vi "test Loopback MC.vi"(8 "error in":errorcluster, 11 "TestCase in":refnum<class "Loopback.lvclass">) -> (0 "error out":errorcluster, 3 "TestCase out":refnum<class "Loopback.lvclass">)   [LabVIEW 2020, in "Loopback.lvclass"]
uses:
  Loopback.lvclass
  C:/dev/niveristand-custom-device-testing-tools/VeriStandTestCase/VeriStandTestCase.lvclass
  <vilib>/numeric/Random Number (Range) U64.vi
  485b7c2b-8320-4722-9ec7-d01f27c65546.vi
  0f9dda61-2c21-4955-8588-a8fc95227647.vi
  <vilib>/numeric/sub_Random U32.vi
  <vilib>/NI VeriStand/Execution/Workspace/NI VeriStand - Set Single Channel Value.vi
  <vilib>/NI VeriStand/Execution/Workspace/NI VeriStand - Get Single Channel Value.vi
  <vilib>/addons/_JKI Toolkits/VI Tester/TestCase.llb/TestCase.lvclass
  <vilib>/NI VeriStand/Execution/Workspace/NI_VS Workspace ExecutionAPI.lvlib
  C:/Program Files (x86)/National Instruments/LabVIEW 2020/vi.lib/addons/_JKI Toolkits/VI Tester/TestCase.llb/TestCase.lvclass
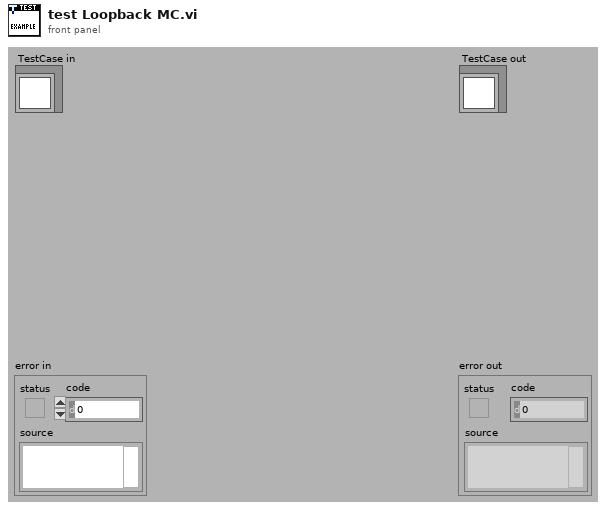
[diagram p1: front panel]
types:
  T1 = typedef "NI_VS Workspace ExecutionAPI.lvlib/WorkspaceAPI.ctl" = refnum<k24>
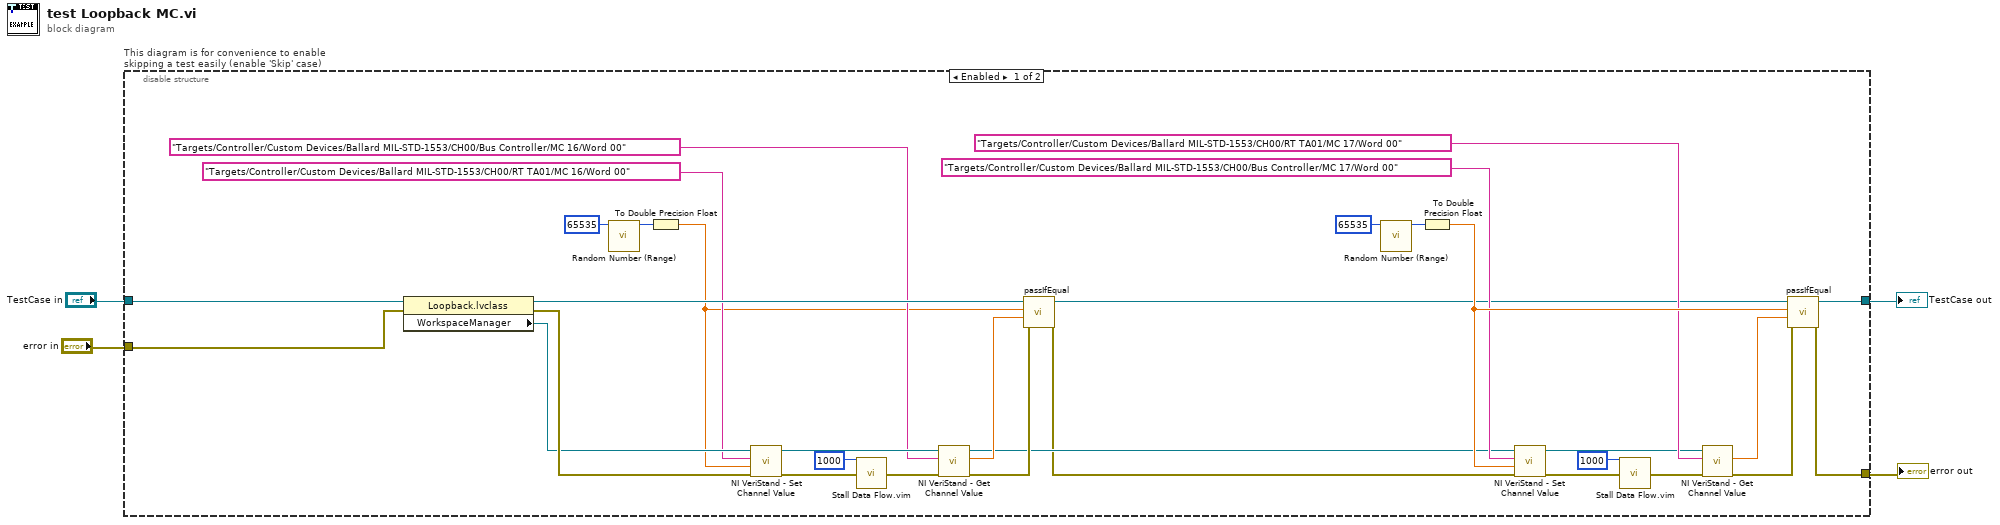
[diagram p0: block diagram]
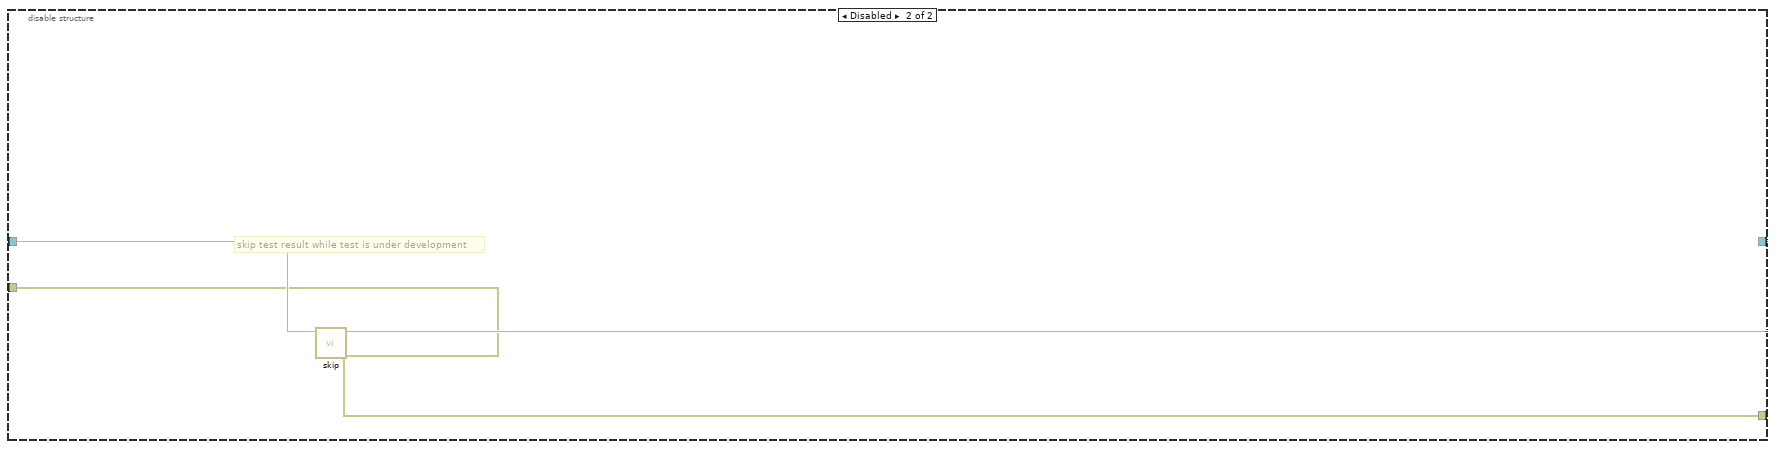
[diagram p2: hidden frame]
diagram:
  n1 = disable-structure "This diagram is for convenience to enable skipping a test easily (enable 'Skip' case)" shown="Enabled" {
    disable-tunnel: "TestCase in" -> [w27 w40]
    disable-tunnel: [w10 w38] -> w1
    disable-tunnel: [w5 w39] -> w3
    disable-tunnel: "error in" -> [w24 w37]
    frame Enabled {
      n2 = property class="Loopback.lvclass"(reference=w27, error in=w24) -> (reference out=w36:refnum<class "Loopback.lvclass">, error out=w31:errorcluster, "WorkspaceManager"=w29:T1)
      n3 = call-poly <vilib>:"Random Number (Range).vi"("upper bound (100)"=u64 65535) -> ("number"=w9:u64)  [unwired: 10 in]
      n4 = To Double Precision Float(number=w9) -> (double precision float=w23:dbl)
      n5 = call-poly <vilib>:"NI VeriStand - Set Channel Value.vi"("error in (no error)"=w31, "Value"=w23, "Channel"="Targets/Controller/Custom Devices/Ballard MIL-STD-1553/CH00/RT TA01/MC 16/Word 00", "WorkspaceManager in"=w29) -> ("error out"=w33:errorcluster, "WorkspaceManager out"=w35:T1)  [unwired: 6 in]
      n6 = call "Stall Data Flow.vim"("value in"=w33, "milliseconds to wait"=u32 1000) -> ("value out"=w34:errorcluster)  [unwired: 1 out]
      n7 = call-poly <vilib>:"NI VeriStand - Get Channel Value.vi"("error in (no error)"=w34, "Channel"="Targets/Controller/Custom Devices/Ballard MIL-STD-1553/CH00/Bus Controller/MC 16/Word 00", "WorkspaceManager in"=w35) -> ("error out"=w30:errorcluster, "Value"=w28:dbl, "WorkspaceManager out"=w12:T1)  [unwired: 6 in]
      n8 = call-dynamic "passIfEqual.vi"("error in (no error)"=w30, "y"=w28, "x"=w23, "TestCase in"=w36) -> ("error out"=w11:errorcluster, "TestCase out"=w13:refnum<class "Loopback.lvclass">)  [unwired: 6 in]
      n9 = call-poly <vilib>:"Random Number (Range).vi"("upper bound (100)"=u64 65535) -> ("number"=w7:u64)  [unwired: 10 in]
      n10 = To Double Precision Float(number=w7) -> (double precision float=w22:dbl)
      n11 = call-poly <vilib>:"NI VeriStand - Set Channel Value.vi"("error in (no error)"=w11, "Value"=w22, "Channel"="Targets/Controller/Custom Devices/Ballard MIL-STD-1553/CH00/Bus Controller/MC 17/Word 00", "WorkspaceManager in"=w12) -> ("error out"=w16:errorcluster, "WorkspaceManager out"=w14:T1)  [unwired: 6 in]
      n12 = call "Stall Data Flow.vim"("value in"=w16, "milliseconds to wait"=u32 1000) -> ("value out"=w15:errorcluster)  [unwired: 1 out]
      n13 = call-poly <vilib>:"NI VeriStand - Get Channel Value.vi"("error in (no error)"=w15, "Channel"="Targets/Controller/Custom Devices/Ballard MIL-STD-1553/CH00/RT TA01/MC 17/Word 00", "WorkspaceManager in"=w14) -> ("error out"=w18:errorcluster, "Value"=w19:dbl)  [unwired: 6 in, 1 out]
      n14 = call-dynamic "passIfEqual.vi"("error in (no error)"=w18, "y"=w19, "x"=w22, "TestCase in"=w13) -> ("error out"=w5:errorcluster, "TestCase out"=w10:refnum<class "Loopback.lvclass">)  [unwired: 6 in]
    }
    frame Disabled {
      # "skip test result while test is under development"
      n15 = call <vilib>:"skip.vi"("error in (no error)"=w37, "TestCase in"=w40) -> ("error out"=w39:errorcluster, "TestCase out"=w38:refnum<class "Loopback.lvclass">)  [unwired: 8 in]
    }
  }
  "error out" <- w3
  "TestCase out" <- w1
